vi "Index_Config.vi"(8 "Action":string, 11 "config":string[][](array[string])) -> (3 "data":string)   [LabVIEW 2017]
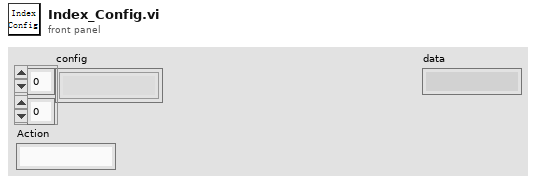
[diagram p1: front panel]
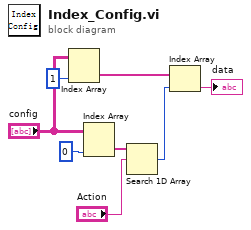
[diagram p0: block diagram]
diagram:
  n1 = Index Array(array="config", index (col)=1 ("禁用的索引 (列)")) -> (element=w4:string[])  [unwired: 1 in]
  n2 = Index Array(array="config", index (col)=0 ("禁用的索引 (列)")) -> (element=w7:string[])  [unwired: 1 in]
  n3 = Search 1D Array(1D array=w7, element="Action") -> (index of element=w3:i32)  [unwired: 1 in]
  n4 = Index Array(array=w4, index=w3) -> (element=→"data":string)
